vi "Dut Tx Initiate.vi"(0 "MTK7615 in":refnum<class "MTK7615.lvclass">, 11 "error in (no error)":errorcluster) -> (4 "MTK7615 out":refnum<class "MTK7615.lvclass">, 15 "error out":errorcluster)   [LabVIEW 2015, in "MTK7615.lvlib" / "MTK7615.lvclass"]
uses:
  MTK7615.lvclass
  MTK7615.lvclass/MTK7615.ctl
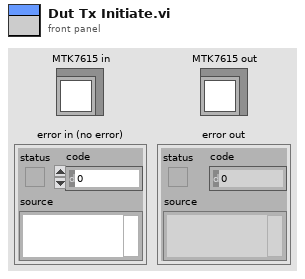
[diagram p1: front panel]
types:
  T1 = typedef "niDCT_TELNET_PrivRef.ctl" = refnum<data-value>
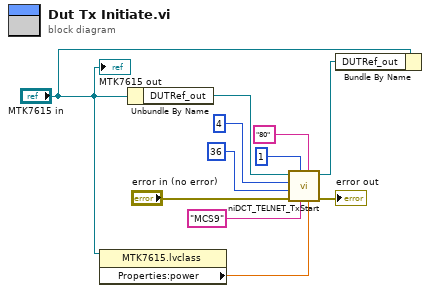
[diagram p0: block diagram]
diagram:
  n1 = property class="MTK7615.lvclass"(reference="MTK7615 in") -> ("Properties:power"=w7:dbl)  [unwired: 1 in, 2 out]
  n2 = Unbundle By Name("MTK7615 in") -> ("DUTRef_out"=w11:T1)
  n3 = call "niDCT_TELNET_TxStart.vi"("TxLevel"=w7, "Bandwidth"="80", "DataRate"="MCS9", "Chain"=1, "error in (no error)"="error in (no error)", "ChannelNumber"=36, "Standard"=4, "DUTRef"=w11) -> ("error out"=→"error out":errorcluster, "DUTRef_out"=w1:T1)  [unwired: 2 in]
  n4 = Bundle By Name(cluster="MTK7615 in", "DUTRef_out"=w1) -> ()  [unwired: 1 out]
  "MTK7615 out" <- "MTK7615 in"
